vi "line follow autonomous.vi"() -> ()   [LabVIEW 2012, in "Omni2013.lvrbt"]
uses:
  Omni2013.lvrbt
  <vilib>/NXT/Hardware/Plugins/Tetrix 180 deg Servo/Tetrix180ServoAddress.ctl
  <vilib>/NXT/Hardware/Plugins/Tetrix DC Motor/TetrixDCMotorAddress.ctl
  <vilib>/NXT/HiTechnic/HiTechnic Controls/HiTechnic Port.ctl
  <vilib>/NXT/Block Support/NXT_InputPort.ctl
  <vilib>/NXT/Dual Mode Library/Waits/Wait_Num(msec).vi
  <vilib>/NXT/NXTIO Xnodes/NXTIONodeSubVIs/TETRIX IO Move Servos.vi
  <vilib>/NXT/NXTIO Xnodes/NXTIONodeSubVIs/TETRIX IO Move DC Motors.vi
  <vilib>/NXT/HiTechnic/HiTechnic Config/HiTechnic IRSeeker Mode1200Hz.vi
  <vilib>/NXT/HiTechnic/HiTechnic SubVIs/HiTechnic IRSeeker Sensor_AC dir.vi
  <vilib>/NXT/Dual Mode Library/Sensors/Sonar_cm.vi
  <vilib>/NXT/Dual Mode Library/Display/drawNumber.vi
  <vilib>/NXT/HiTechnic/HiTechnic Read/HiTechnic IRSeeker Sensor_DC all.vi
  <vilib>/NXT/Dual Mode Library/Sensors/Light_On.vi
  <vilib>/NXT/NXTIO Xnodes/AddressXNode/NXTIOAddress.xnode
  <vilib>/NXT/NXTIO Xnodes/NXTIOXNode/NXTIO.xnode
  <vilib>/NXT/Subs/LVHSConnector.ctl
  <vilib>/NXT/LegoClasses/BrickReference/BrickReference.lvclass
panel:
  in  "Translation U&D 2":dbl
  in  "Translation L&R 2":dbl
  in  "Initial Time":dbl
  in  "Translation U&D":dbl
  in  "Translation L&R":dbl
  in  "Rotation":dbl
  out "Enabled":bool
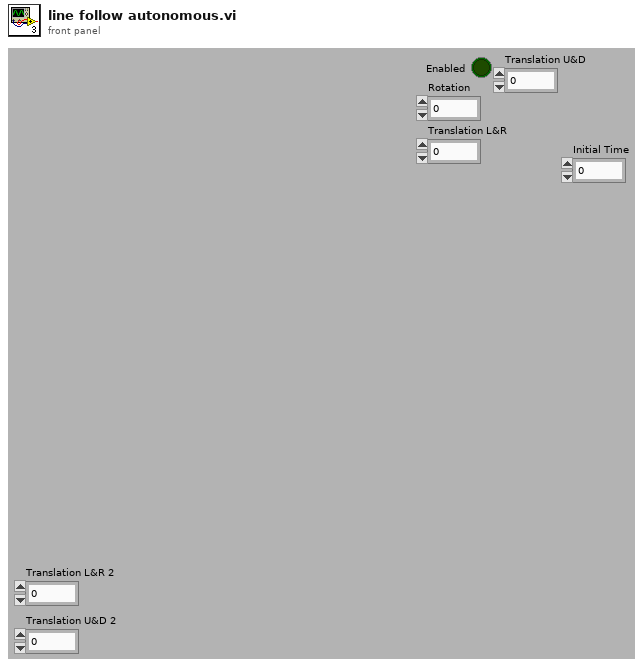
[diagram p1: front panel]
types:
  T1 = typedef "LVHSConnector.ctl" = refnum<class "BrickReference.lvclass">
  T2 = typedef "HiTechnic Port.ctl" = cluster{"Port":T3, "MUX Port":u8}
  T3 = typedef "NXT_InputPort.ctl" = u8
  T4 = typedef "TetrixDCMotorAddress.ctl" = i16
  T5 = cluster{"TetrixDCMotor":T4, "TetrixDCMotor 2":T4}
  T6 = typedef "Tetrix180ServoAddress.ctl" = i16
  T7 = cluster{"Direction (0-9)":i16, "Signal Strength (Array)":u8[]}
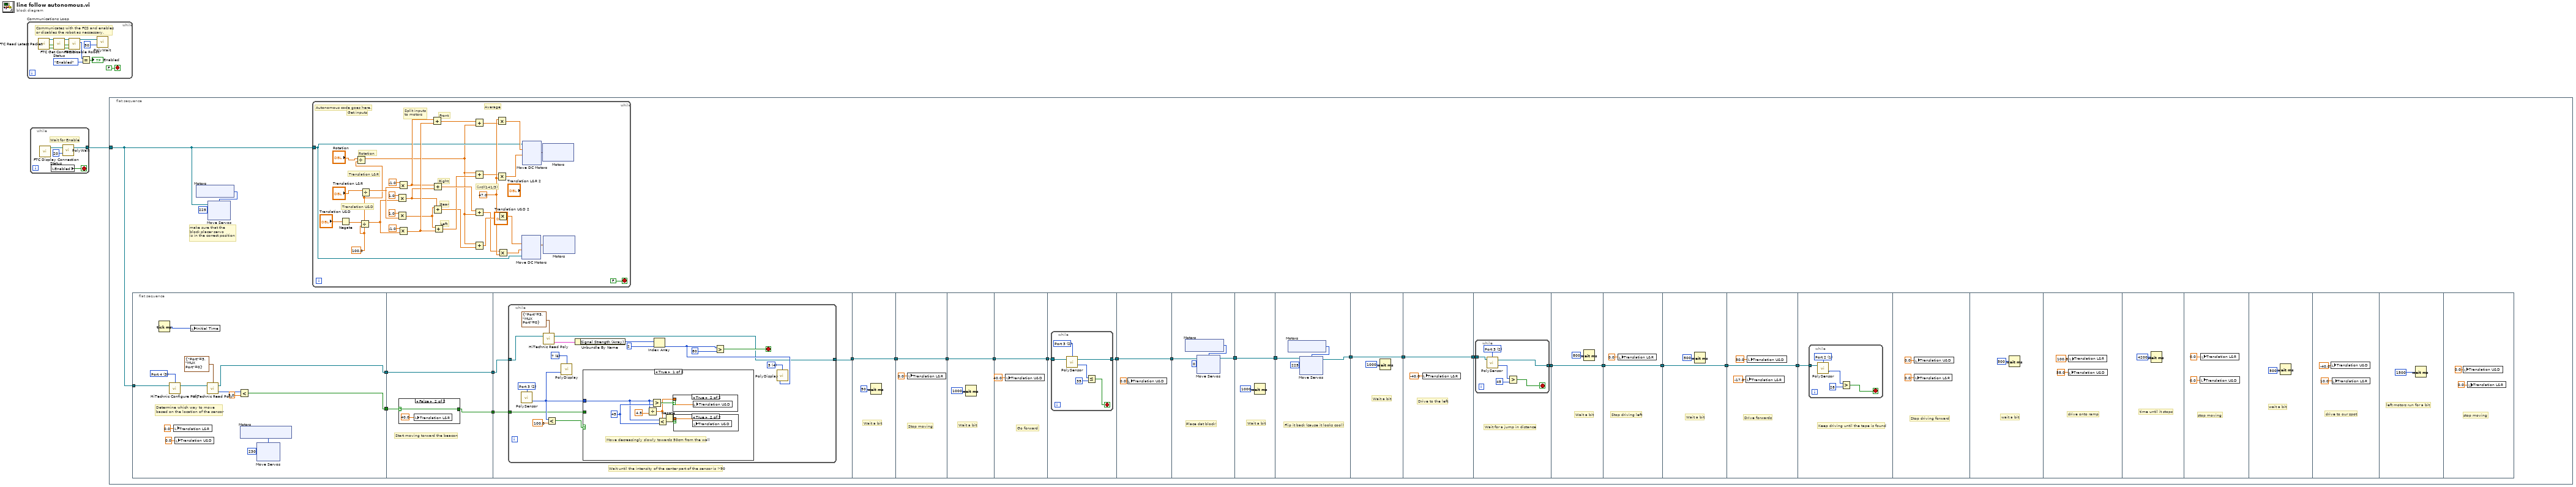
[diagram p0: block diagram]
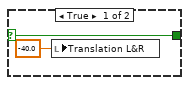
[diagram p2: hidden frame]
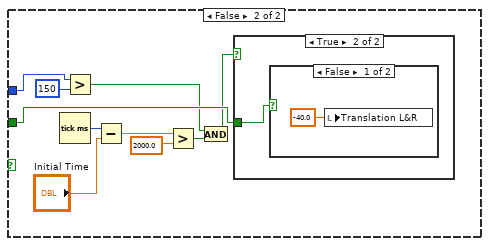
[diagram p5: hidden frame]
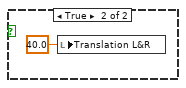
[diagram p7: hidden frame]
diagram:
  n1 = while "Communications Loop" {
    stop <- FALSE stop-if-true
    # "Communicates with the FCS and enables \nor disables the robot as neccessary."
    n2 = call <vilib>:"FTC Read Latest Packet.vi"() -> ("Packet Received?"=w11:bool, "Stopped?"=w10:bool, "NXT"=w13:T1)  [unwired: 6 in, 3 out]
    n3 = call <vilib>:"FTC Get Connection Status.vi"("Packet Received?"=w11, "Stopped?"=w10, "NXT"=w13) -> ("Online?"=w2:bool, "Stopped?"=w3:bool, "NXT"=w12:T1)  [unwired: 5 in]
    n4 = call <vilib>:"FTC Disable Robot.vi"("Online?"=w2, "Stopped?"=w3, "NXT"=w12) -> ("Enabled?"=w6:enum16{"Disabled", "Enabled"}, "NXT"=w8:T1)  [unwired: 3 in]
    n5 = Equal?(x=w6, y=enum16{"Disabled", "Enabled"}."Enabled") -> (x = y?=→"Enabled":bool)
    n6 = call-poly <vilib>:"PolyWait.vi"("Time (100 msec)"=u32 50 ("Time (msec)"), "NXT"=w8) -> ()  [unwired: 2 in, 1 out]
  }
  n7 = while {
    tunnel: [w15] -> w1
    stop <- w16 stop-if-true
    # "Wait for Enable"
    n8 = call <vilib>:"FTC Display Connection Status.vi"() -> ("NXT"=w14:T1)  [unwired: 11 in]
    n9 = local read "Enabled"() -> (w16:bool)
    n10 = call-poly <vilib>:"PolyWait.vi"("Time (100 msec)"=u32 20 ("Time (msec)"), "NXT"=w14) -> ("NXT"=w15:T1)  [unwired: 2 in]
  }
  n11 = flat-sequence {
    tunnel: w1 -> [w39]
    frame #0 {
      # "make sure that the \nblock placer servo \nis in the correct position"
      n12 = flat-sequence {
        tunnel: [w50] -> w28
        tunnel: [w51] -> w27
        tunnel: w39 -> [w56]
        tunnel: [w73] -> w36
        tunnel: w28 -> [w72]
        tunnel: w27 -> [w73]
        tunnel: [w71] -> w26
        tunnel: w36 -> [w80]
        tunnel: [w79] -> w38
        tunnel: w26 -> [w78]
        tunnel: w38 -> [w120]
        tunnel: [w120] -> w37
        tunnel: [w121] -> w35
        tunnel: w37 -> [w121]
        tunnel: [w124] -> w29
        tunnel: w35 -> [w124]
        tunnel: w29 -> [w126]
        tunnel: [w126] -> w34
        tunnel: w34 -> [w128]
        tunnel: [w127] -> w33
        tunnel: w33 -> [w136]
        tunnel: [w136] -> w32
        tunnel: w32 -> [w138]
        tunnel: [w137] -> w31
        tunnel: w31 -> [w150]
        tunnel: [w150] -> w30
        tunnel: w30 -> [w152]
        tunnel: [w151] -> w23
        tunnel: [w163] -> w24
        tunnel: w23 -> [w163]
        tunnel: [w165] -> w25
        tunnel: w24 -> [w165]
        tunnel: w25 -> [w168]
        tunnel: [w167] -> w18
        tunnel: [w175] -> w19
        tunnel: w18 -> [w175]
        tunnel: [w177] -> w20
        tunnel: w19 -> [w177]
        tunnel: [w179] -> w21
        tunnel: w20 -> [w179]
        tunnel: [w181] -> w22
        tunnel: w21 -> [w181]
        tunnel: w22 -> [w184]
        frame #0 {
          w59 = T3 3 items=["Port 1", "Port 2", "Port 3", "Port 4"] ("Port")
          # "Determine which way to move \nbased on the location of the sensor"
          n13 = Tick Count (ms)() -> (millisecond timer value=w55:u32)
          n14 = call-poly <vilib>:"HiTechnic Configure Poly.vi"("NXT"=w56, "Port"=w59) -> ("NXT"=w60:T1)  [unwired: 2 in]
          n15 = local write "Translation L&R"(0.0 ("Translation L&R")) -> ()
          n16 = local write "Translation U&D"(0.0 ("Translation U&D")) -> ()
          n17 = local write "Initial Time"(w55) -> ()
          n18 = call-poly <vilib>:"HiTechnic Read Poly.vi"("NXT"=w60, "Port/MUX"=T2 {"Port"=3, "MUX Port"=0}) -> ("Direction (0-9)"=w54:i16, "NXT"=w51:T1)  [unwired: 1 in]
          n19 = Less?(x=w54, y=5.0) -> (x < y?=w50:bool)
          n20 = xnode "Motors"() -> ("Motor"=w53:T6)
          n21 = xnode "Move Servos"("Position 1"=u8 230, "Servos"=w53) -> ()  [unwired: 1 in, 1 out]
        }
        frame #1 {
          # "Start moving torward the beacon"
          n22 = case shown="False" w72 {
            selector: w72 -> [w74 w76]
            tunnel: [w74 w76] -> w71
            frame True {
              n23 = local write "Translation L&R"(-40.0 ("Translation L&R")) -> ()
            }
            frame False {
              n24 = local write "Translation L&R"(40.0 ("Translation L&R")) -> ()
            }
          }
        }
        frame #2 {
          # "Wait until the intensity of the center part of the sensor is >90"
          n25 = while {
            tunnel: w80 -> [w88]
            tunnel: [w86] -> w79
            tunnel: w78 -> [w81]
            stop <- w92 stop-if-true
            w85 = i16 6 items=["1", "2", "3", "4", "5", "6", "7", "8"] ("Line")
            w87 = T3 2 items=["Port 1", "Port 2", "Port 3", "Port 4"] ("Port (Port 4)")
            w91 = i16 4 items=["1", "2", "3", "4", "5", "6", "7", "8"] ("Line")
            n26 = call-poly <vilib>:"PolySensor.vi"("Port (Port 4)"=w87) -> ("Distance (cm)"=w83:i16)  [unwired: 2 in, 1 out]
            n27 = call-poly <vilib>:"HiTechnic Read Poly.vi"("NXT"=w88, "Port/MUX"=T2 {"Port"=3, "MUX Port"=0}) -> ("All Info"=w95:T7, "NXT"=w86:T1)  [unwired: 1 in]
            n28 = Less?(x=w83, y=100.0) -> (x < y?=w82:bool)
            n29 = call-poly <vilib>:"PolyDisplay.vi"("number"=w83, "Line"=w85) -> ()  [unwired: 2 in, 1 out]
            n30 = Unbundle By Name(w95) -> ("Signal Strength (Array)"=w94:u8[])
            n31 = case shown="True" w82 {
              tunnel: w83 -> [w99 w115]
              tunnel: w81 -> [_ w113]
              frame True {
                w101 = i16 45 ("y")
                # "Move decreasingly slowly towards 50cm from the wall"
                n32 = Divide(x=w99, y=4.5) -> (x/y=w98:dbl)
                n33 = Greater?(x=w99, y=w101) -> (0:w102:bool)
                n34 = Less?(x=w99, y=w101) -> (x < y?=w103:bool)
                n35 = Negate(x=w98) -> (-x=w97:dbl)
                n36 = case shown="True" w102 {
                  tunnel: w98 -> [_ w104]
                  frame False {
                  }
                  frame True {
                    n37 = local write "Translation U&D"(w104) -> ()
                  }
                }
                n38 = case shown="True" w103 {
                  tunnel: w97 -> [_ w105]
                  frame False {
                  }
                  frame True {
                    n39 = local write "Translation U&D"(w105) -> ()
                  }
                }
              }
              frame False {
                n40 = Tick Count (ms)() -> (millisecond timer value=w112:u32)
                n41 = Greater?(x=w115, y=i16 150) -> (0:w107:bool)
                n42 = Subtract(x=w112, y="Initial Time") -> (x-y=w110:dbl)
                n43 = Greater?(x=w110, y=2000.0) -> (0:w106:bool)
                n44 = And(x=w107, y=w106) -> (x .and. y?=w108:bool)
                n45 = case shown="True" w108 {
                  tunnel: w113 -> [_ w116]
                  frame False {
                  }
                  frame True {
                    n46 = case shown="False" w116 {
                      frame False {
                        n47 = local write "Translation L&R"(-40.0 ("Translation L&R")) -> ()
                      }
                      frame True {
                        n48 = local write "Translation L&R"(40.0 ("Translation L&R")) -> ()
                      }
                    }
                  }
                }
              }
            }
            n49 = Index Array(array=w94, index=2) -> (element=w90:u8)
            n50 = Greater?(x=w90, y=u8 80) -> (0:w92:bool)
            n51 = call-poly <vilib>:"PolyDisplay.vi"("number"=w90, "Line"=w91) -> ()  [unwired: 2 in, 1 out]
          }
        }
        frame #3 {
          # "Wait a bit"
          n52 = Wait (ms)(milliseconds to wait=u32 50) -> ()  [unwired: 1 out]
        }
        frame #4 {
          # "Stop moving"
          n53 = local write "Translation L&R"(0.0 ("Translation L&R")) -> ()
        }
        frame #5 {
          # "Wait a bit"
          n54 = Wait (ms)(milliseconds to wait=u32 1000) -> ()  [unwired: 1 out]
        }
        frame #6 {
          # "Go forward"
          n55 = local write "Translation U&D"(40.0 ("Translation U&D")) -> ()
        }
        frame #7 {
          n56 = while {
            tunnel: w128 -> [w131]
            tunnel: [w130] -> w127
            stop <- w132 stop-if-true
            w129 = T3 2 items=["Port 1", "Port 2", "Port 3", "Port 4"] ("Port (Port 4)")
            n57 = call-poly <vilib>:"PolySensor.vi"("NXT"=w131, "Port (Port 4)"=w129) -> ("Distance (cm)"=w134:i16, "NXT"=w130:T1)  [unwired: 1 in]
            n58 = Less Or Equal?(x=w134, y=i16 35) -> (x <= y?=w132:bool)
          }
        }
        frame #8 {
          n59 = local write "Translation U&D"(0.0 ("Translation U&D")) -> ()
        }
        frame #9 {
          # "Place dat block!"
          n60 = xnode "Motors"() -> ("Motor"=w140:T6)
          n61 = xnode "Move Servos"("Position 1"=u8 0, "Servos"=w140, "NXT"=w138) -> ("NXT"=w137:T1)
        }
        frame #10 {
          # "Wait a bit"
          n62 = Wait (ms)(milliseconds to wait=u32 1000) -> ()  [unwired: 1 out]
        }
        frame #11 {
          # "Flip it back (cause it looks cool)"
          n63 = xnode "Motors"() -> ("Motor"=w154:T6)
          n64 = xnode "Move Servos"("Position 1"=u8 225, "Servos"=w154, "NXT"=w152) -> ("NXT"=w151:T1)
        }
        frame #12 {
          # "Wait a bit"
          n65 = Wait (ms)(milliseconds to wait=u32 1000) -> ()  [unwired: 1 out]
        }
        frame #13 {
          # "Drive to the left"
          n66 = local write "Translation L&R"(-40.0 ("Translation L&R")) -> ()
        }
        frame #14 {
          # "Wait for a jump in distance"
          n67 = while {
            tunnel: w168 -> [w170]
            tunnel: [w169] -> w167
            stop <- w172 stop-if-true
            w174 = T3 2 items=["Port 1", "Port 2", "Port 3", "Port 4"] ("Port (Port 4)")
            n68 = call-poly <vilib>:"PolySensor.vi"("NXT"=w170, "Port (Port 4)"=w174) -> ("Distance (cm)"=w171:i16, "NXT"=w169:T1)  [unwired: 1 in]
            n69 = Greater?(x=w171, y=i16 45) -> (0:w172:bool)
          }
        }
        frame #15 {
          # "Wait a bit"
          n70 = Wait (ms)(milliseconds to wait=u32 800) -> ()  [unwired: 1 out]
        }
        frame #16 {
          # "Stop driving left"
          n71 = local write "Translation L&R"(0.0 ("Translation L&R")) -> ()
        }
        frame #17 {
          # "Wait a bit"
          n72 = Wait (ms)(milliseconds to wait=u32 500) -> ()  [unwired: 1 out]
        }
        frame #18 {
          # "Drive forwards"
          n73 = local write "Translation L&R"(-17.0 ("Translation L&R")) -> ()
          n74 = local write "Translation U&D"(30.0 ("Translation U&D")) -> ()
        }
        frame #19 {
          # "Keep driving until the tape is found"
          n75 = while {
            tunnel: w184 -> [w185]
            stop <- w188 stop-if-true
            w187 = T3 1 items=["Port 1", "Port 2", "Port 3", "Port 4"] ("Port (Port 3)")
            n76 = call-poly <vilib>:"PolySensor.vi"("NXT"=w185, "Port (Port 3)"=w187) -> ("Scaled Value"=w186:i16)  [unwired: 1 in, 1 out]
            n77 = Greater?(x=w186, y=i16 28) -> (0:w188:bool)
          }
        }
        frame #20 {
          # "Stop driving forward"
          n78 = local write "Translation L&R"(0.0 ("Translation L&R")) -> ()
          n79 = local write "Translation U&D"(0.0 ("Translation U&D")) -> ()
        }
        frame #21 {
          # "wait a bit"
          n80 = Wait (ms)(milliseconds to wait=u32 500) -> ()  [unwired: 1 out]
        }
        frame #22 {
          # "drive onto ramp"
          n81 = local write "Translation U&D"(58.0 ("Translation U&D")) -> ()
          n82 = local write "Translation L&R"(100.0 ("Translation L&R")) -> ()
        }
        frame #23 {
          # "time until it stops"
          n83 = Wait (ms)(milliseconds to wait=u32 4200) -> ()  [unwired: 1 out]
        }
        frame #24 {
          # "stop moving"
          n84 = local write "Translation U&D"(0.0 ("Translation U&D")) -> ()
          n85 = local write "Translation L&R"(0.0 ("Translation L&R")) -> ()
        }
        frame #25 {
          # "wait a bit"
          n86 = Wait (ms)(milliseconds to wait=u32 500 ("millisecond timer value")) -> ()  [unwired: 1 out]
        }
        frame #26 {
          # "drive to our spot"
          n87 = local write "Translation U&D"(-40.0 ("Translation U&D")) -> ()
          n88 = local write "Translation L&R"(10.0 ("Translation L&R")) -> ()
        }
        frame #27 {
          # "left motors run for a bit"
          n89 = Wait (ms)(milliseconds to wait=u32 1500 ("millisecond timer value")) -> ()  [unwired: 1 out]
        }
        frame #28 {
          # "stop moving"
          n90 = local write "Translation U&D"(0.0 ("Translation U&D")) -> ()
          n91 = local write "Translation L&R"(0.0 ("Translation L&R")) -> ()
        }
      }
      n92 = xnode "Motors"() -> ("Motor"=w41:T6)
      n93 = xnode "Move Servos"("Position 1"=u8 225, "Servos"=w41, "NXT"=w39) -> ()  [unwired: 1 out]
      n94 = while {
        tunnel: w39 -> [w209]
        stop <- FALSE stop-if-true
        w205 = 100.0 ("y")
        w236 = 47.0 ("y")
        # "Average"
        # "Left"
        # "Rear"
        # "Right"
        # "Front"
        # "(int)(141/3)"
        # "Split inputs to motors"
        # "Get inputs"
        # "Translation U&D"
        # "Rotation"
        # "Translation L&R"
        # "Autonomous code goes here."
        n95 = Negate(x="Translation U&D") -> (-x=w204:dbl)
        n96 = Divide(x="Rotation", y=w205) -> (x/y=w206:dbl)
        n97 = Divide(x=w204, y=w205) -> (x/y=w207:dbl)
        n98 = Divide(x="Translation L&R", y=w205) -> (x/y=w208:dbl)
        n99 = Multiply(x=1.0, y=w207) -> (x*y=w230:dbl)
        n100 = Multiply(x=1.0, y=w208) -> (x*y=w219:dbl)
        n101 = Multiply(x=-1.0, y=w208) -> (x*y=w218:dbl)
        n102 = Multiply(x=-1.0, y=w207) -> (x*y=w231:dbl)
        n103 = Add(x=w218, y=w231) -> (x+y=w215:dbl)
        n104 = Add(x=w218, y=w230) -> (x+y=w217:dbl)
        n105 = Add(x=w219, y=w230) -> (x+y=w214:dbl)
        n106 = Add(x=w219, y=w231) -> (x+y=w216:dbl)
        n107 = Add(x=w215, y=w206) -> (x+y=w234:dbl)
        n108 = Add(x=w206, y=w216) -> (x+y=w233:dbl)
        n109 = Add(x=w217, y=w206) -> (x+y=w232:dbl)
        n110 = Add(x=w206, y=w214) -> (x+y=w235:dbl)
        n111 = Multiply(x=w236, y=w234) -> (x*y=w225:dbl)
        n112 = Multiply(x=w233, y=w236) -> (x*y=w226:dbl)
        n113 = Multiply(x=w236, y=w235) -> (x*y=w229:dbl)
        n114 = Multiply(x=w232, y=w236) -> (x*y=w228:dbl)
        n115 = xnode "Motors"() -> ("Motor"=w224:cluster{"TetrixDCMotor":T4, "TetrixDCMotor":T4})
        n116 = xnode "Move DC Motors"("Power/Speed 2"=w226, "Power/Speed 1"=w225, "Motors"=w224, "NXT"=w209) -> ()  [unwired: 1 out]
        n117 = xnode "Motors"() -> ("Motor"=w227:cluster{"TetrixDCMotor":T4, "TetrixDCMotor":T4})
        n118 = xnode "Move DC Motors"("Power/Speed 2"=w228, "Power/Speed 1"=w229, "Motors"=w227, "NXT"=w209) -> ()  [unwired: 1 out]
      }
    }
  }
